vi "Actor Core.vi"(8 "error in":errorcluster, 11 "Sweeper  in":refnum<class "Sweeper.lvclass">) -> (0 "error out":errorcluster, 3 "Actor out":refnum<class "Actor.lvclass">)   [LabVIEW 2015, in "Sweeper.lvclass"]
doc: "(<B>Filename</B>: Actor Framework.lvlib:Actor.lvclass:Actor Core.vi)\n\nReceives messages to the actor, reacts to them, and initiates any error handling that may shut the actor down.\n\nDescendant classes may override this VI to append parallel tasks for the actor to complete while it handles messages. Overrides use the Call Parent Method node."
uses:
  Sweeper.lvclass
  <vilib>/ActorFramework/Actor/Actor.lvclass
  NHMFL_Core/Libraries/Instruments/Instrument Driver/Sweeper Driver/Sweep Configuration.ctl
  Measure_core/Instrument Recorders/Instrument Recorder/Instrument Recorder.lvclass
panel:
  in  "Configuration":T1 {"Sweep  rate" format="%#_6p"; "End sweep" format="%#_6p"; "Start sweep" format="%#_6p"}
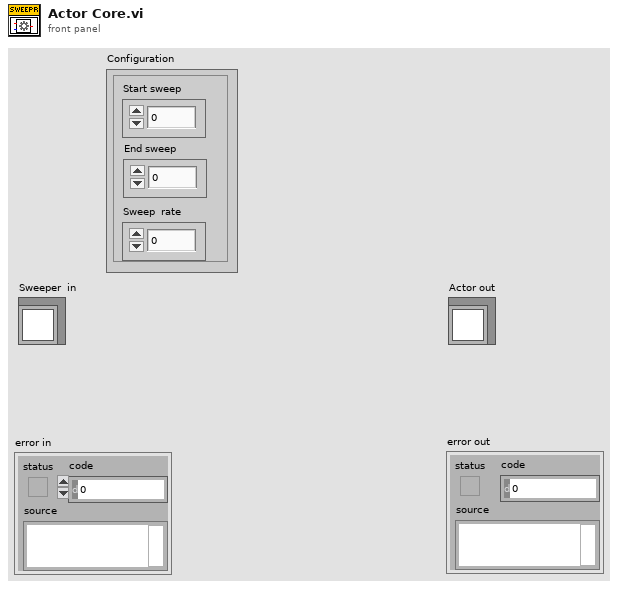
[diagram p1: front panel]
types:
  T1 = typedef "Sweep Configuration.ctl" = cluster{"Start sweep":dbl, "End sweep":dbl, "Sweep  rate":dbl}
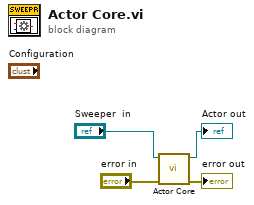
[diagram p0: block diagram]
diagram:
  n1 = call-parent "Actor Core.vi"("error in"="error in", "Measure Object in"="Sweeper  in") -> ("error out"=→"error out":errorcluster, "Actor out"=→"Actor out":refnum<class "Actor.lvclass">)  [unwired: 8 in]
